vi "Make From Packed Library.vi"(10 "Fully Qualified String":string) -> (2 "Fully Qualified String out":string)   [LabVIEW 2017, in "Composition.lvlib"]
doc: "Changes \".lvlib\" to \".lvlibp\" if the first part of the fully qualified string refers to \".lvlib\". Otherwise, it returns the original string."
uses:
  Composition.lvlib
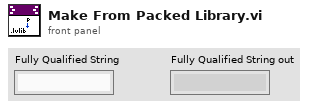
[diagram p1: front panel]
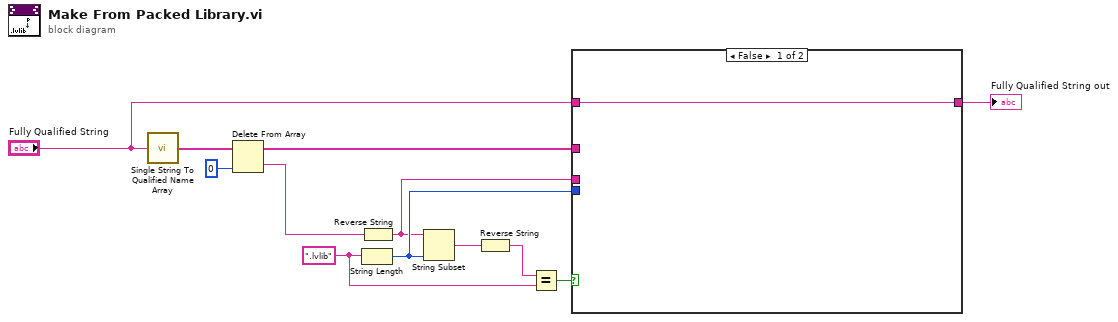
[diagram p0: block diagram]
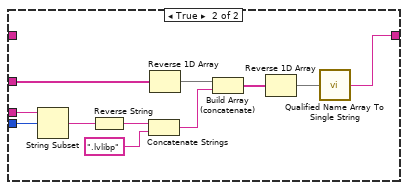
[diagram p2: hidden frame]
diagram:
  w9 = ".lvlib"
  n1 = call <vilib>:"Single String To Qualified Name Array.vi"("Fully Qualified String"="Fully Qualified String") -> ("Fully Qualified Array"=w8:string[])
  n2 = Delete From Array(array=w8, index=0) -> (deleted portion=w5:string, array with subset deleted=w4:string[])  [unwired: 1 in]
  n3 = String Length(string=w9) -> (length=w7:i32)
  n4 = Reverse String(1:w5) -> (0:w6:string)
  n5 = String Subset(string=w6, length (rest)=w7) -> (substring=w11:string)  [unwired: 1 in]
  n6 = Reverse String(1:w11) -> (0:w10:string)
  n7 = Equal?(x=w10, y=w9) -> (x = y?=w3:bool)
  n8 = case shown="False" w3 {
    tunnel: w7 -> [_ w21]
    tunnel: w6 -> [_ w20]
    tunnel: w4 -> [_ w19]
    tunnel: "Fully Qualified String" -> [w13 _]
    tunnel: [w13 w14] -> w1
    frame False {
    }
    frame True {
      n9 = String Subset(string=w20, offset (0)=w21) -> (substring=w24:string)  [unwired: 1 in]
      n10 = Reverse String(1:w24) -> (0:w23:string)
      n11 = Concatenate Strings(w23, ".lvlibp" ("string")) -> (w16:string)
      n12 = Reverse 1D Array(array=w19) -> (reversed array=w18:string[])
      n13 = Build Array (concatenate)(w18, w16) -> (w17:string[])
      n14 = Reverse 1D Array(array=w17) -> (reversed array=w15:string[])
      n15 = call <vilib>:"Qualified Name Array To Single String.vi"("Fully Qualified Array"=w15) -> ("Fully Qualified String"=w14:string)
    }
  }
  "Fully Qualified String out" <- w1
